vi "stepper generic.vi"(5 "wait until positon":bool, 7 "motor":T1(ring), 8 "error in (no error) 2":errorcluster, 9 "move to":dbl=1.0 min=-193273528.32 max=193273528.0 step=0.09 format="%.2f", 10 "menu":enum16{"read step", "move"}(ring), 11 "Instrument Address":refnum<visa-resource-name>) -> (0 "error out":errorcluster, 3 "read value":dbl)   [LabVIEW 2021]
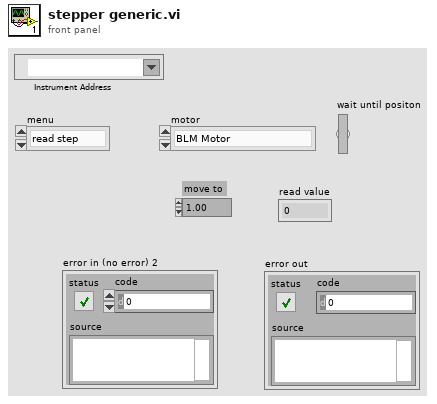
[diagram p1: front panel]
types:
  T1 = enum16{"BLM Motor", "IMS Motor", "Generic stepper motor"}
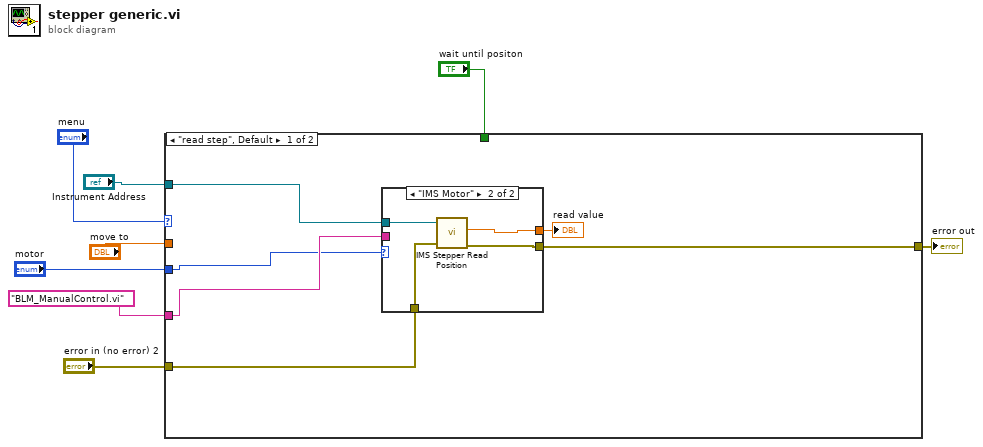
[diagram p0: block diagram]
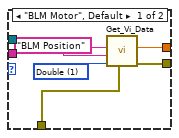
[diagram p2: hidden frame]
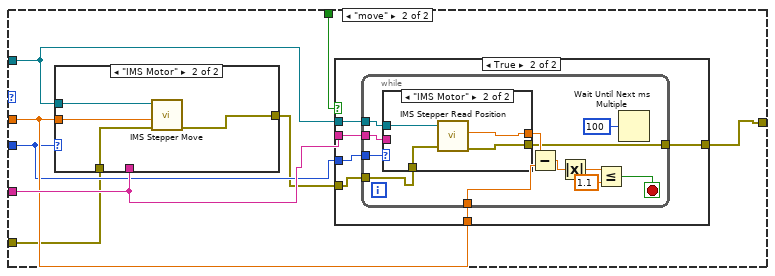
[diagram p3: hidden frame]
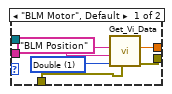
[diagram p5: hidden frame]
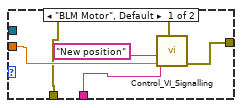
[diagram p6: hidden frame]
diagram:
  n1 = case shown="\"read step\", Default" "menu" {
    tunnel: "Instrument Address" -> [w14 w28]
    tunnel: "move to" -> [_ w30]
    tunnel: "wait until positon" -> [_ w32]
    tunnel: "BLM_ManualControl.vi" ("Target VI name") -> [w13 w31]
    tunnel: "motor" -> [w11 w29]
    tunnel: "error in (no error) 2" -> [w10 w27]
    tunnel: [w9 w25] -> w1
    frame "read step", Default {
      n2 = case shown="\"IMS Motor\"" w11 {
        tunnel: w13 -> [w19 _]
        tunnel: [w17 w23] -> w12
        tunnel: w14 -> [_ w24]
        tunnel: w10 -> [w16 w21]
        tunnel: [w15 w22] -> w9
        frame "BLM Motor", Default {
          w18 = u16 1 items=["String", "Double", "Boolean", "Variant"] ("Data Type")
          n3 = call "Get_Vi_Data.vi"("error in (no error) 2"=w16, "Data Type"=w18, "VI name"=w19, "Control Name"="BLM Position") -> ("error out"=w15:errorcluster, "Data (Double)"=w17:dbl)  [unwired: 3 in, 3 out]
        }
        frame "IMS Motor" {
          n4 = call "IMS Stepper Read Position.vi"("Instrument Address"=w24, "error in (no error)"=w21) -> ("Response"=w23:dbl, "error out"=w22:errorcluster)  [unwired: 2 in, 1 out]
        }
      }
      "read value" <- w12
    }
    frame "move" {
      n5 = case shown="\"IMS Motor\"" w29 {
        tunnel: w28 -> [_ w70]
        tunnel: w30 -> [w65 w69]
        tunnel: w31 -> [w64 _]
        tunnel: w27 -> [w63 w68]
        tunnel: [w62 w67] -> w26
        frame "BLM Motor", Default {
          n6 = call "Control_VI_Signalling.vi"("error in (no error)"=w63, "Input Value"=w65, "Control Name"="New position", "Target VI name"=w64) -> ("error out"=w62:errorcluster)  [unwired: 7 in]
        }
        frame "IMS Motor" {
          n7 = call "IMS Stepper Move.vi"("error in (no error)"=w68, "Distance"=w69, "Instrument Address"=w70) -> ("error out"=w67:errorcluster)  [unwired: 4 in, 1 out]
        }
      }
      n8 = case shown="True" w32 {
        tunnel: w31 -> [_ w39]
        tunnel: w30 -> [_ w38]
        tunnel: w29 -> [_ w37]
        tunnel: w28 -> [_ w36]
        tunnel: w26 -> [w33 w35]
        tunnel: [w33 w34] -> w25
        frame False {
        }
        frame True {
          n9 = while {
            tunnel: w39 -> [w51]
            tunnel: w38 -> [w49]
            tunnel: w37 -> [w43]
            tunnel: w36 -> [w42]
            tunnel: w35 -> [w41]
            tunnel: [w40] -> w34
            stop <- w45 stop-if-true
            n10 = case shown="\"IMS Motor\"" w43 {
              tunnel: w51 -> [w56 _]
              tunnel: [w54 w60] -> w50
              tunnel: w42 -> [_ w61]
              tunnel: w41 -> [w52 w59]
              tunnel: [w53 w58] -> w40
              frame "BLM Motor", Default {
                w55 = u16 1 items=["String", "Double", "Boolean", "Variant"] ("Data Type")
                n11 = call "Get_Vi_Data.vi"("error in (no error) 2"=w52, "Data Type"=w55, "VI name"=w56, "Control Name"="BLM Position") -> ("error out"=w53:errorcluster, "Data (Double)"=w54:dbl)  [unwired: 3 in, 3 out]
              }
              frame "IMS Motor" {
                n12 = call "IMS Stepper Read Position.vi"("Instrument Address"=w61, "error in (no error)"=w59) -> ("Response"=w60:dbl, "error out"=w58:errorcluster)  [unwired: 2 in, 1 out]
              }
            }
            n13 = Subtract(x=w50, y=w49) -> (x-y=w48:dbl)
            n14 = Absolute Value(x=w48) -> (abs(x)=w47:dbl)
            n15 = Less Or Equal?(x=w47, y=1.1) -> (x <= y?=w45:bool)
            n16 = Wait Until Next ms Multiple(millisecond multiple=u32 100) -> ()  [unwired: 1 out]
          }
        }
      }
    }
  }
  "error out" <- w1
